vi "machine_vision.vi"() -> ()   [LabVIEW 2017]
uses:
  controls/State.ctl
  <vilib>/Utility/error.llb/DialogType.ctl
  <vilib>/express/express analysis/Spectral/Block/exnSpectralBlock spectral measurements RMS poly.vi
  <vilib>/express/express analysis/Spectral/Block/exnSpectralBlock spectral measurements RMS WFM.vi
  <vilib>/express/express analysis/Spectral/XNode/ExpressSpectralMeasurementsBlockNode.xnode
panel:
  in  "File name for saving":path=path "test.dat" caption="Filename"
  in  "File directory for saving":path=path "C:/Users/LAB_SPT/Desktop" caption="Filename"
  in  "Rate, samples/sec":dbl=100000.0 min=0.0 max=1000000.0 step=1.0 format="%#_6p"
  in  "Write Button":bool
  out "Fourier Spectrum":cluster{"f0":dbl, "df":dbl, "magnitude":dbl[]}(graph)={"f0"=0.0, "df"=0.0001, "magnitude"=array[5000 elements]}
  out "Aquired Signal":dynamicdata(graph)=[{"t0"=timestamp(3595315136.41372 s since 1904-01-01), "dt"=9.999999999999972e-06, "Y"=array[10000 elements], "attributes"=variant("NI_ChannelName"=variant(string "Voltage_0"), "NI_UnitDescription"=variant(string "Volts"))}] caption="Waveform Graph 2"
  in  "Device Aquire Signal":tag="DAQ_6363"
  out "Sawtooth Signal":dynamicdata(graph)=[{"t0"=timestamp(3595315136.4137154 s since 1904-01-01), "dt"=9.999999999999972e-06, "Y"=array[10000 elements], "attributes"=variant("NI_ChannelName"=variant(string "Voltage"), "NI_UnitDescription"=variant(string "Volts"))}]
  in  "Device Sawtooth Signal Generation":tag="DAQ_6363"
  out "error out":errorcluster
  in  "Number of Samples to read":i32=10000 min=1 step=1 format="%.0p"
  in  "Error In (no error)":errorcluster
  in  "Exit Button":bool
  out "Status":string="Off"
  # "Если выскакивает ошибка, просто запустить программу заново"
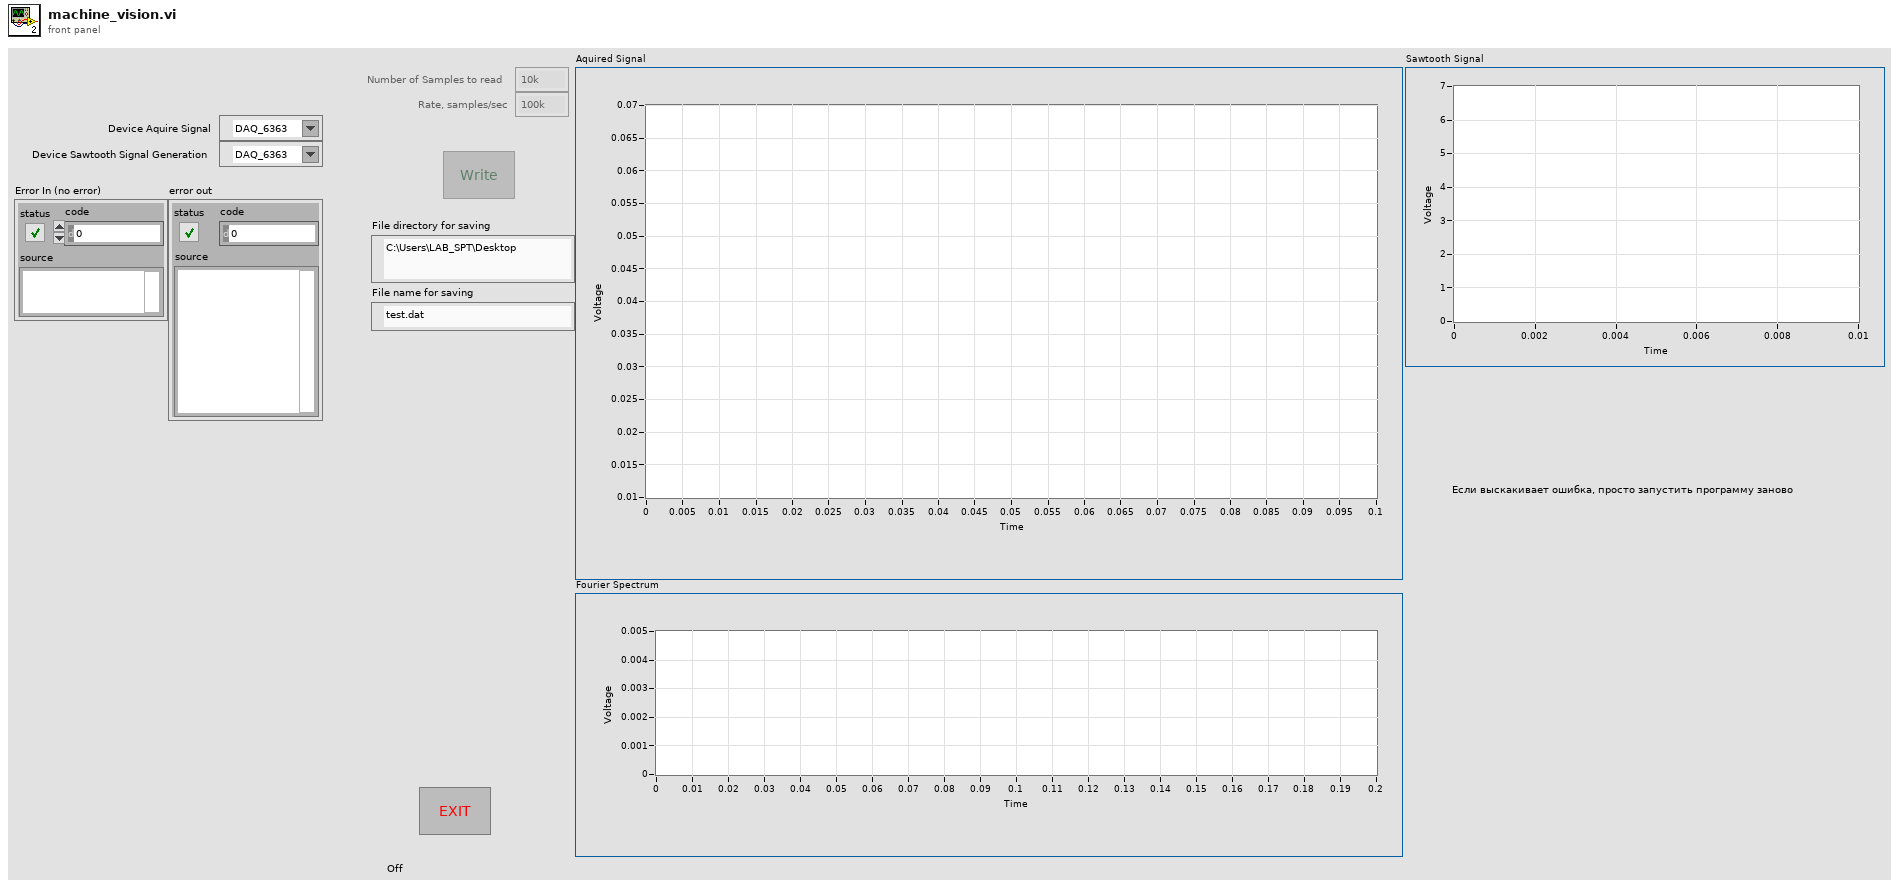
[diagram p1: front panel]
types:
  T1 = typedef "State.ctl" = enum16{"Init", "Idle", "Shutdown"}
  T2 = cluster{"averaging mode":u16, "weighting mode":u16, "number of averages":u32}
  T3 = cluster{"dB On (F)":bool, "unwrap phase (F)":bool, "convert to degree (F)":bool}
  T4 = typedef "DialogType.ctl" = u16
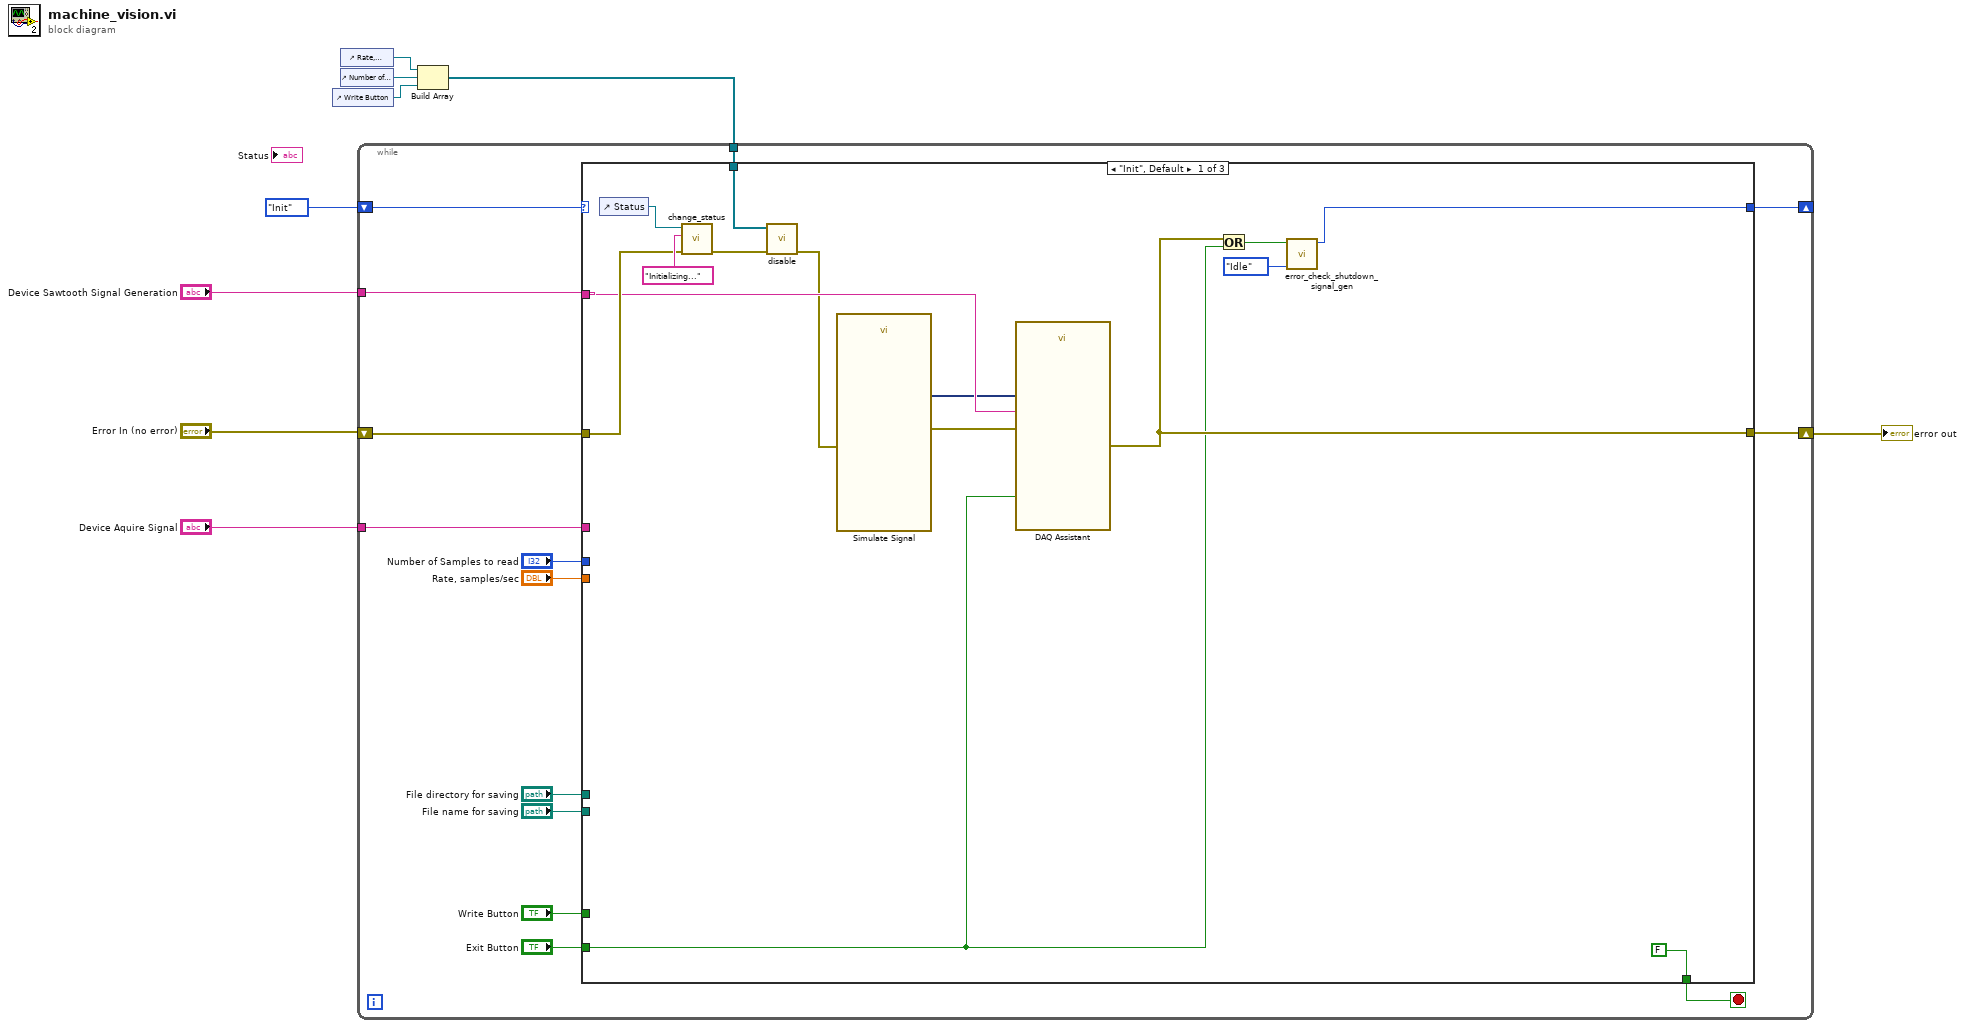
[diagram p0: block diagram]
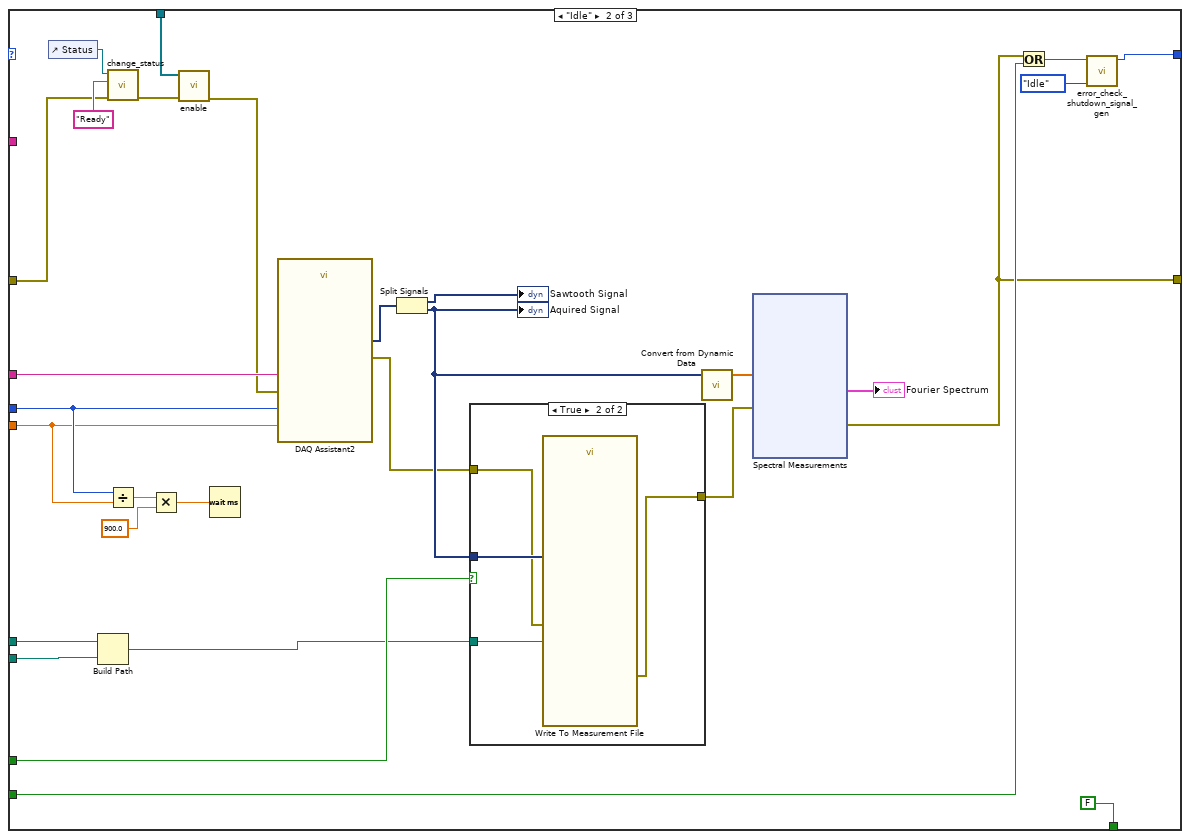
[diagram p2: hidden frame]
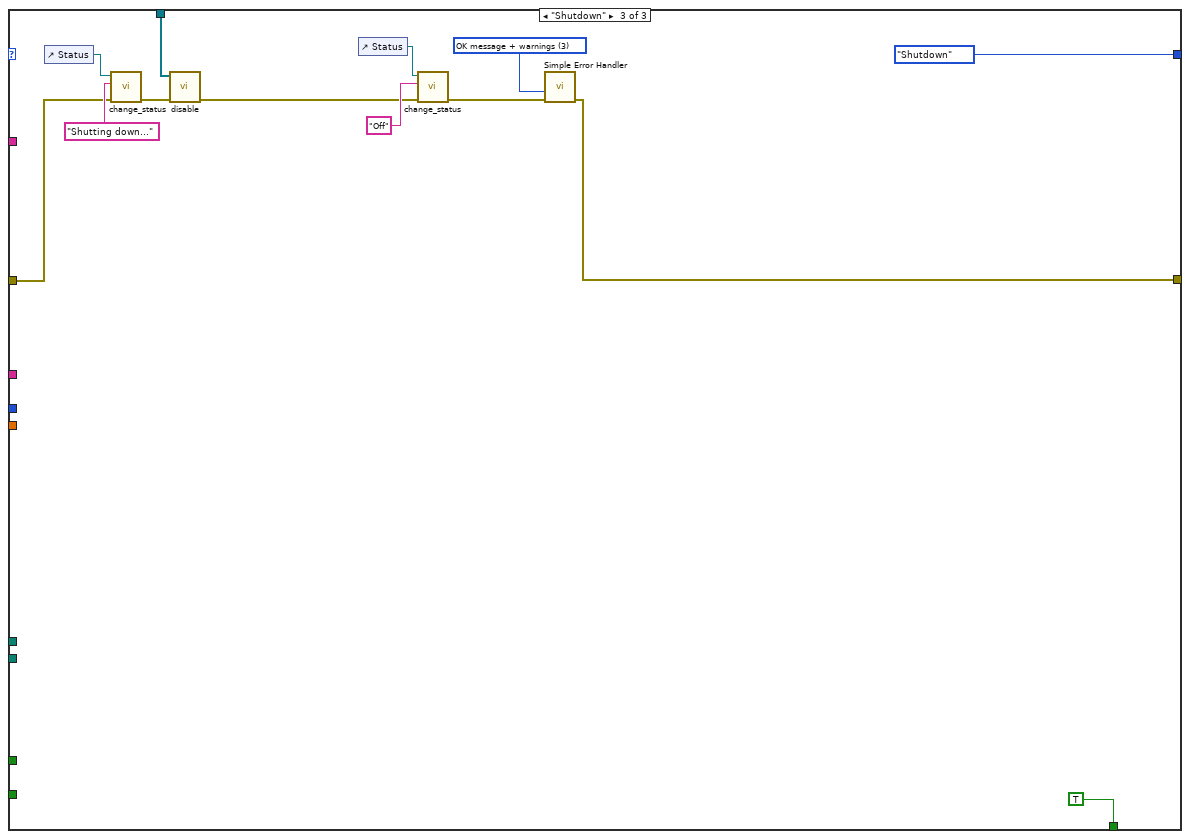
[diagram p4: hidden frame]
diagram:
  n1 = control-ref of="Write Button"() -> (w1:refnum<vi>)
  n2 = control-ref of="Rate, samples/sec"() -> (w2:refnum<vi>)
  n3 = control-ref of="Number of Samples to read"() -> (w6:refnum<vi>)
  n4 = Build Array(w2, w6, w1) -> (w8:refnum<vi>[])
  n5 = while {
    shift-right: [w20] -> _
    shift-left: State."Init" -> [w23]
    shift-right: [w19] -> w7
    shift-left: "Error In (no error)" -> [w21]
    tunnel: w8 -> [w17]
    tunnel: "Device Sawtooth Signal Generation" -> [w15]
    tunnel: "Device Aquire Signal" -> [w14]
    stop <- w16 stop-if-true
    n6 = case shown="\"Init\", Default" w23 {
      tunnel: "Exit Button" -> [w24 w58 _]
      tunnel: w21 -> [w35 w65 w92]
      tunnel: [w32 w62 State."Shutdown" ("State Out")] -> w20
      tunnel: [w27 w50 w88] -> w19
      tunnel: "Number of Samples to read" -> [_ w46 _]
      tunnel: w17 -> [w25 w60 w83]
      tunnel: [FALSE FALSE TRUE] -> w16
      tunnel: w15 -> [w30 _ _]
      tunnel: w14 -> [_ w59 _]
      tunnel: "Write Button" -> [_ w49 _]
      tunnel: "Rate, samples/sec" -> [_ w45 _]
      tunnel: "File directory for saving" -> [_ w41 _]
      tunnel: "File name for saving" -> [_ w40 _]
      frame "Init", Default {
        n7 = control-ref of="Status"() -> (w36:refnum<vi>)
        n8 = call "change_status.vi"("error in (no error)"=w35, "String"="Initializing...", "String in"=w36) -> ("error out"=w38:errorcluster)  [unwired: 8 in]
        n9 = call "disable.vi"("error in (no error)"=w38, "Array"=w25) -> ("error out"=w26:errorcluster)  [unwired: 9 in]
        n10 = call "Simulate Signal"("error in (no error)"=w26) -> ("Sawtooth"=w28:dynamicdata, "error out"=w29:errorcluster)  [unwired: 13 in]
        n11 = call "DAQ Assistant"("data"=w28, "error in"=w29, "stop (F)"=w24, "device name"=w30) -> ("error out"=w27:errorcluster)  [unwired: 13 in, 2 out]
        n12 = Or(x=w27, y=w24) -> (x .or. y?=w34:bool)
        n13 = call "error_check_shutdown_signal_gen.vi"("State In"=State."Idle", "Boolean"=w34) -> ("State Out"=w32:T1)  [unwired: 9 in]
      }
      frame "Idle" {
        n14 = control-ref of="Status"() -> (w67:refnum<vi>)
        n15 = Build Path(base path=w41, name or relative path=w40) -> (appended path=w39:path)
        n16 = call "change_status.vi"("error in (no error)"=w65, "String"="Ready", "String in"=w67) -> ("error out"=w48:errorcluster)  [unwired: 8 in]
        n17 = Divide(x=w46, y=w45) -> (x/y=w44:dbl)
        n18 = Multiply(x=w44, y=900.0) -> (x*y=w42:dbl)
        n19 = call "enable.vi"("error in (no error)"=w48, "Array"=w60) -> ("error out"=w47:errorcluster)  [unwired: 9 in]
        n20 = Wait (ms)(milliseconds to wait=w42) -> ()  [unwired: 1 out]
        n21 = call "DAQ Assistant2"("rate"=w45, "number of samples"=w46, "error in"=w47, "device name"=w59) -> ("data"=w57:dynamicdata, "error out"=w52:errorcluster)  [unwired: 12 in, 2 out]
        n22 = Split Signals(w57) -> (→"Sawtooth Signal":dynamicdata, w53:dynamicdata)  [unwired: 2 in]
        "Aquired Signal" <- w53
        n23 = case shown="True" w49 {
          tunnel: w53 -> [_ w72]
          tunnel: w52 -> [w68 w71]
          tunnel: [w68 w70] -> w51
          tunnel: w39 -> [_ w69]
          frame False {
          }
          frame True {
            n24 = call "Write To Measurement File"("Signals"=w72, "error in (no error)"=w71, "Filename"=w69) -> ("error out"=w70:errorcluster)  [unwired: 14 in, 2 out]
          }
        }
        n25 = call "Convert from Dynamic Data"("Dynamic Data Type"=w53) -> ("Array"=w55:dbl[])  [unwired: 3 in]
        n26 = xnode "Spectral Measurements"("Signals"=w55, "error in (no error)"=w51) -> ("FFT - (RMS)"=→"Fourier Spectrum":cluster{"f0":dbl, "df":dbl, "magnitude":dbl[]}, "error out"=w50:errorcluster)  [unwired: 1 out]
        n27 = Or(x=w50, y=w58) -> (x .or. y?=w64:bool)
        n28 = call "error_check_shutdown_signal_gen.vi"("State In"=State."Idle", "Boolean"=w64) -> ("State Out"=w62:T1)  [unwired: 9 in]
      }
      frame "Shutdown" {
        w90 = T4 3 items=["no dialog", "OK message", "continue or stop message", "OK message + warnings", "continue/stop + warnings"] ("type of dialog (OK msg:1)")
        n29 = control-ref of="Status"() -> (w95:refnum<vi>)
        n30 = call "change_status.vi"("error in (no error)"=w92, "String"="Shutting down...", "String in"=w95) -> ("error out"=w93:errorcluster)  [unwired: 8 in]
        n31 = call "disable.vi"("error in (no error)"=w93, "Array"=w83) -> ("error out"=w84:errorcluster)  [unwired: 9 in]
        n32 = control-ref of="Status"() -> (w86:refnum<vi>)
        n33 = call "change_status.vi"("error in (no error)"=w84, "String"="Off", "String in"=w86) -> ("error out"=w87:errorcluster)  [unwired: 8 in]
        n34 = call <vilib>:"Simple Error Handler.vi"("type of dialog (OK msg:1)"=w90, "error in (no error)"=w87) -> ("error out"=w88:errorcluster)  [unwired: 3 in, 4 out]
      }
    }
  }
  "error out" <- w7
